vi "ETH8_E2L_Checksum.vi"(11 "unsigned byte array":u8[](array[numeric])) -> (3 "Checksum":bool)   [LabVIEW 2022 SP3]
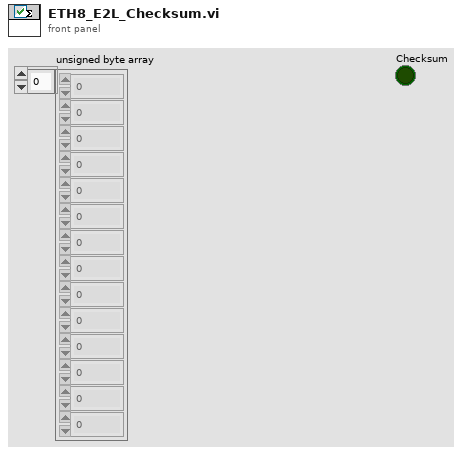
[diagram p1: front panel]
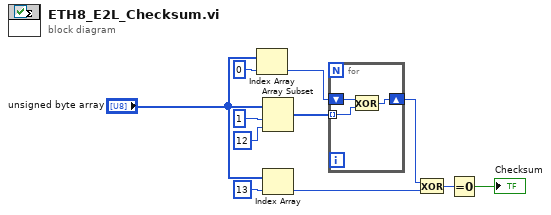
[diagram p0: block diagram]
diagram:
  n1 = Index Array(array="unsigned byte array", index=0) -> (element=w9:u8)
  n2 = Array Subset(array="unsigned byte array", index=1 ("length"), length=12 ("index")) -> (w10:u8[])
  n3 = Index Array(array="unsigned byte array", index=13) -> (element=w4:u8)
  n4 = for {
    shift-right: [w12] -> w5
    shift-left: w9 -> [w14]
    tunnel: w10 -> [w13] mode=indexing
    n5 = Exclusive Or(1:w13, 2:w14) -> (0:w12:u8)
  }
  n6 = Exclusive Or(1:w4, 2:w5) -> (0:w3:u8)
  n7 = Equal To 0?(x=w3) -> (x = 0?=→"Checksum":bool)
